vi "State_Machine.vi"(0 "Path In":path, 1 "Emergency":bool, 2 "Start Process":bool, 3 "Initialized":bool, 4 "Input Validated":bool, 5 "error in (no error)":errorcluster, 6 "Action":enum16{""}(ring), 7 "Running Done":bool, 9 "Process Complete":bool, 11 "Progressing":bool, 12 "Reset":bool, 13 "Powering Down":bool) -> (14 "Path Out":path, 15 "State":dbl, 16 "State String":string, 19 "error out":errorcluster)   [LabVIEW 2018]
panel:
  in  "Empty 2":bool
  in  "Empty1":bool
  out "_C_Powering_Down":bool
  out "_C_Empty_2":bool
  out "_C_Start_Process":bool
  out "_C_Empty_1":bool
  out "_C_Progressing":bool
  out "_C_Process Complete":bool
  out "_C_Running_Done":bool
  out "_C_Input_Validated":bool
  out "_C_Initialized":bool
  out "_C_emergency":bool
  out "_Powering Down":bool
  out "_Progressing Stage":bool
  out "_Completing Stage":bool
  out "_Running Stage":bool
  out "_Validating Input":bool
  out "_Initializing":bool
  out "_Idle":bool
  out "_Emergency":bool
  out "_Current_State":dbl
  # "~~~STATE MACHINE OUTPUT KEY~~~\n~~~ 1x Numeric & 1x Boolean ~~~\n(neg) - Emergency\n   All negative values\n(max) - Powering Down\n   All values above max\n0 -Idle\n1 - Initializing\n2 - Validating Input\n3 - Running Stage\n4 - Completing Stage\n5 - Progressing Stage\nBoolean - (T/F) Emergency Status"
  # "~~~INPUT CONDITIONS KEY~~~\n~~~ x10 Boolean Values~~~\n1 - Emergency\n2 - Start Process\n3 - Initialized\n4 - Input Validated\n5 - Running Done\n6 - Process Complete\n7 - Progressing (To next stage)\n8 - (Empty 1)\n9 - (Empty 2)\n10 - Powering Down"
  # "Local Variables (Used For Debugging)"
  # "State Lights"
  # "Condition Lights"
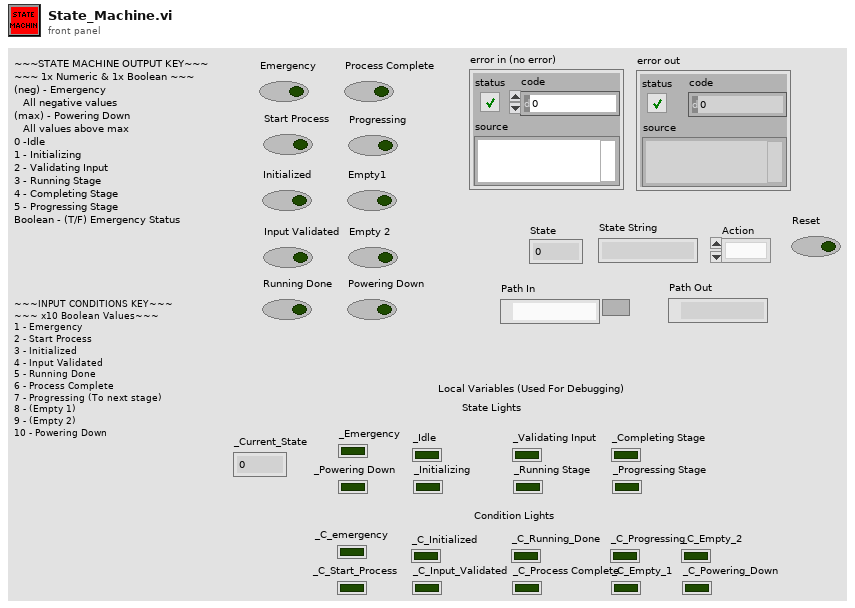
[diagram p1: front panel]
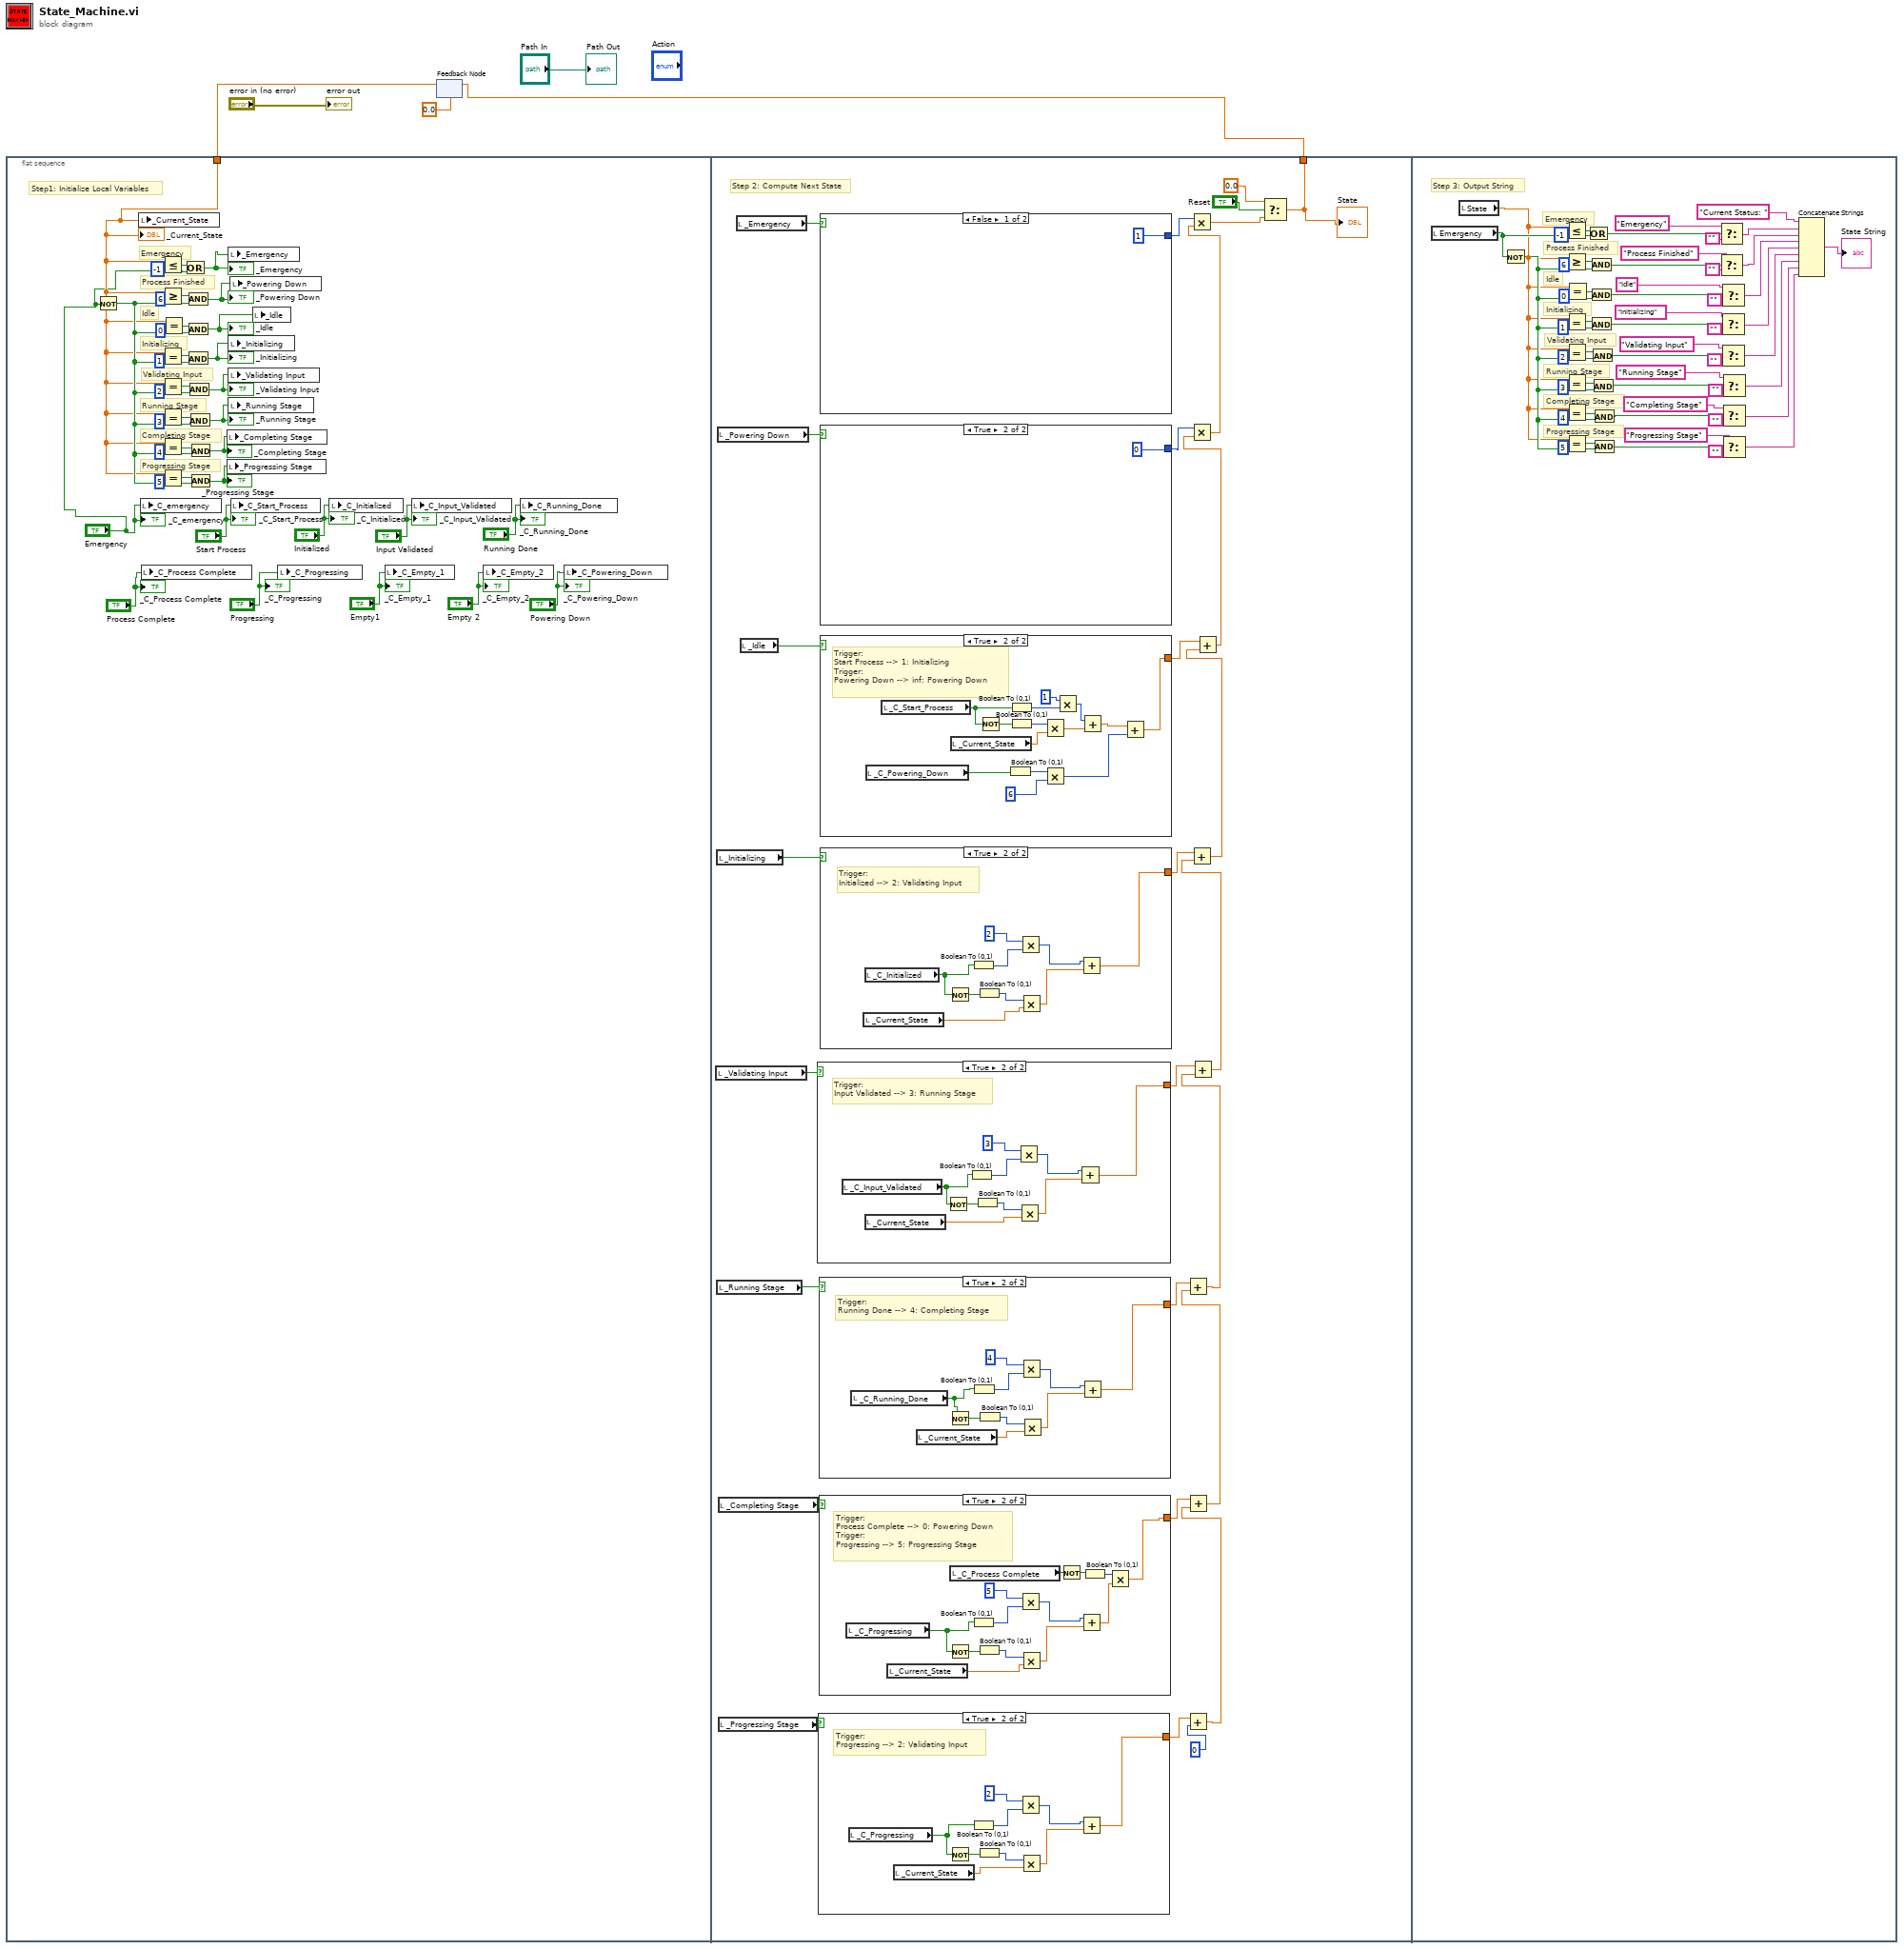
[diagram p0: block diagram]
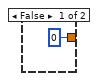
[diagram p2: hidden frame]
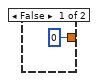
[diagram p3: hidden frame]
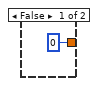
[diagram p4: hidden frame]
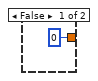
[diagram p5: hidden frame]
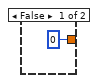
[diagram p6: hidden frame]
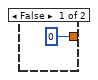
[diagram p7: hidden frame]
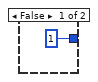
[diagram p8: hidden frame]
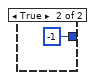
[diagram p9: hidden frame]
diagram:
  n1 = flat-sequence {
    tunnel: w4 -> [w16]
    tunnel: [w42] -> w1
    frame #0 {
      # "Step1: Initialize Local Variables"
      # "Emergency"
      # "Process Finished"
      # "Progressing Stage"
      # "Completing Stage"
      # "Running Stage"
      # "Validating Input"
      # "Initializing"
      # "Idle"
      n2 = Not(x="Emergency") -> (.not. x?=w30:bool)
      n3 = local write "_Current_State"(w16) -> ()
      n4 = local write "_C_emergency"("Emergency") -> ()
      n5 = local write "_C_Process Complete"("Process Complete") -> ()
      n6 = Less Or Equal?(x=w16, y=-1) -> (x <= y?=w19:bool)
      n7 = Greater Or Equal?(x=w16, y=6) -> (x >= y?=w17:bool)
      n8 = Equal?(x=w16, y=1) -> (x = y?=w32:bool)
      n9 = Equal?(x=w16, y=2) -> (x = y?=w33:bool)
      n10 = Equal?(x=w16, y=3) -> (x = y?=w34:bool)
      n11 = Equal?(x=w16, y=4) -> (x = y?=w35:bool)
      n12 = Equal?(x=w16, y=5) -> (x = y?=w21:bool)
      n13 = Equal?(x=w16, y=0) -> (x = y?=w31:bool)
      n14 = Or(x=w19, y="Emergency") -> (x .or. y?=w29:bool)
      "_Emergency" <- w29
      n15 = And(x=w17, y=w30) -> (x .and. y?=w28:bool)
      "_Powering Down" <- w28
      n16 = And(x=w31, y=w30) -> (x .and. y?=w27:bool)
      "_Idle" <- w27
      n17 = And(x=w32, y=w30) -> (x .and. y?=w26:bool)
      "_Initializing" <- w26
      n18 = And(x=w33, y=w30) -> (x .and. y?=w25:bool)
      "_Validating Input" <- w25
      n19 = And(x=w34, y=w30) -> (x .and. y?=w24:bool)
      "_Running Stage" <- w24
      n20 = And(x=w35, y=w30) -> (x .and. y?=w23:bool)
      "_Completing Stage" <- w23
      n21 = And(x=w21, y=w30) -> (x .and. y?=w22:bool)
      "_Progressing Stage" <- w22
      n22 = local write "_Completing Stage"(w23) -> ()
      n23 = local write "_Progressing Stage"(w22) -> ()
      n24 = local write "_Emergency"(w29) -> ()
      n25 = local write "_Initializing"(w26) -> ()
      n26 = local write "_Validating Input"(w25) -> ()
      n27 = local write "_Running Stage"(w24) -> ()
      n28 = local write "_Powering Down"(w28) -> ()
      n29 = local write "_C_Start_Process"("Start Process") -> ()
      n30 = local write "_Idle"(w27) -> ()
      n31 = local write "_C_Progressing"("Progressing") -> ()
      n32 = local write "_C_Initialized"("Initialized") -> ()
      n33 = local write "_C_Empty_1"("Empty1") -> ()
      n34 = local write "_C_Input_Validated"("Input Validated") -> ()
      n35 = local write "_C_Empty_2"("Empty 2") -> ()
      n36 = local write "_C_Running_Done"("Running Done") -> ()
      n37 = local write "_C_Powering_Down"("Powering Down") -> ()
      "_Current_State" <- w16
      "_C_emergency" <- "Emergency"
      "_C_Initialized" <- "Initialized"
      "_C_Input_Validated" <- "Input Validated"
      "_C_Running_Done" <- "Running Done"
      "_C_Process Complete" <- "Process Complete"
      "_C_Progressing" <- "Progressing"
      "_C_Empty_1" <- "Empty1"
      "_C_Start_Process" <- "Start Process"
      "_C_Empty_2" <- "Empty 2"
      "_C_Powering_Down" <- "Powering Down"
    }
    frame #1 {
      # "Step 2: Compute Next State"
      n38 = local read "_Validating Input"() -> (w65:bool)
      n39 = local read "_Initializing"() -> (w66:bool)
      n40 = local read "_Running Stage"() -> (w64:bool)
      n41 = local read "_Powering Down"() -> (w68:bool)
      n42 = local read "_Completing Stage"() -> (w63:bool)
      n43 = local read "_Progressing Stage"() -> (w62:bool)
      n44 = local read "_Emergency"() -> (w69:bool)
      n45 = local read "_Idle"() -> (w67:bool)
      n46 = case shown="True" w65 {
        tunnel: [0 w105] -> w52
        frame False {
        }
        frame True {
          # "Trigger:\nInput Validated --> 3: Running Stage"
          n47 = local read "_C_Input_Validated"() -> (w107:bool)
          n48 = local read "_Current_State"() -> (w106:dbl)
          n49 = Not(x=w107) -> (.not. x?=w113:bool)
          n50 = Boolean To (0,1)(Boolean=w107) -> (0, 1=w111:i16)
          n51 = Boolean To (0,1)(Boolean=w113) -> (0, 1=w110:i16)
          n52 = Multiply(x=3, y=w111) -> (x*y=w108:i32)
          n53 = Multiply(x=w110, y=w106) -> (x*y=w109:dbl)
          n54 = Add(x=w108, y=w109) -> (x+y=w105:dbl)
        }
      }
      n55 = case shown="True" w62 {
        tunnel: [0 w71] -> w49
        frame False {
        }
        frame True {
          # "Trigger:\nProgressing --> 2: Validating Input"
          n56 = local read "_C_Progressing"() -> (w73:bool)
          n57 = local read "_Current_State"() -> (w72:dbl)
          n58 = Not(x=w73) -> (.not. x?=w79:bool)
          n59 = Boolean To (0,1)(Boolean=w73) -> (0, 1=w77:i16)
          n60 = Boolean To (0,1)(Boolean=w79) -> (0, 1=w76:i16)
          n61 = Multiply(x=2, y=w77) -> (x*y=w74:i32)
          n62 = Multiply(x=w76, y=w72) -> (x*y=w75:dbl)
          n63 = Add(x=w74, y=w75) -> (x+y=w71:dbl)
        }
      }
      n64 = case shown="True" w64 {
        tunnel: [0 w95] -> w51
        frame False {
        }
        frame True {
          # "Trigger:\nRunning Done --> 4: Completing Stage"
          n65 = local read "_C_Running_Done"() -> (w97:bool)
          n66 = local read "_Current_State"() -> (w96:dbl)
          n67 = Not(x=w97) -> (.not. x?=w103:bool)
          n68 = Boolean To (0,1)(Boolean=w97) -> (0, 1=w101:i16)
          n69 = Boolean To (0,1)(Boolean=w103) -> (0, 1=w100:i16)
          n70 = Multiply(x=4, y=w101) -> (x*y=w98:i32)
          n71 = Multiply(x=w100, y=w96) -> (x*y=w99:dbl)
          n72 = Add(x=w98, y=w99) -> (x+y=w95:dbl)
        }
      }
      n73 = case shown="True" w63 {
        tunnel: [0 w86] -> w50
        frame False {
        }
        frame True {
          # "Trigger:\nProcess Complete --> 0: Powering Down\nTrigger:\nProgressing --> 5: Progressing Stage"
          n74 = local read "_C_Progressing"() -> (w85:bool)
          n75 = local read "_Current_State"() -> (w84:dbl)
          n76 = Not(x=w85) -> (.not. x?=w93:bool)
          n77 = local read "_C_Process Complete"() -> (w83:bool)
          n78 = Boolean To (0,1)(Boolean=w85) -> (0, 1=w91:i16)
          n79 = Boolean To (0,1)(Boolean=w93) -> (0, 1=w90:i16)
          n80 = Multiply(x=5, y=w91) -> (x*y=w88:i32)
          n81 = Multiply(x=w90, y=w84) -> (x*y=w89:dbl)
          n82 = Not(x=w83) -> (.not. x?=w82:bool)
          n83 = Add(x=w88, y=w89) -> (x+y=w87:dbl)
          n84 = Boolean To (0,1)(Boolean=w82) -> (0, 1=w81:i16)
          n85 = Multiply(x=w81, y=w87) -> (x*y=w86:dbl)
        }
      }
      n86 = case shown="False" w69 {
        tunnel: [1 -1] -> w61
        frame False {
        }
        frame True {
        }
      }
      n87 = case shown="True" w68 {
        tunnel: [1 0] -> w46
        frame False {
        }
        frame True {
        }
      }
      n88 = case shown="True" w67 {
        tunnel: [0 w130] -> w54
        frame False {
        }
        frame True {
          # "Trigger:\nStart Process --> 1: Initializing\nTrigger:\nPowering Down --> inf: Powering Down"
          n89 = local read "_C_Powering_Down"() -> (w128:bool)
          n90 = local read "_C_Start_Process"() -> (w137:bool)
          n91 = local read "_Current_State"() -> (w134:dbl)
          n92 = Not(x=w137) -> (.not. x?=w138:bool)
          n93 = Boolean To (0,1)(Boolean=w128) -> (0, 1=w127:i16)
          n94 = Boolean To (0,1)(Boolean=w137) -> (0, 1=w135:i16)
          n95 = Boolean To (0,1)(Boolean=w138) -> (0, 1=w133:i16)
          n96 = Multiply(x=w133, y=w134) -> (x*y=w132:dbl)
          n97 = Multiply(x=w127, y=6) -> (x*y=w125:i32)
          n98 = Multiply(x=1, y=w135) -> (x*y=w131:i32)
          n99 = Add(x=w131, y=w132) -> (x+y=w129:dbl)
          n100 = Add(x=w129, y=w125) -> (x+y=w130:dbl)
        }
      }
      n101 = case shown="True" w66 {
        tunnel: [0 w115] -> w53
        frame False {
        }
        frame True {
          # "Trigger:\nInitialized --> 2: Validating Input"
          n102 = local read "_Current_State"() -> (w117:dbl)
          n103 = local read "_C_Initialized"() -> (w116:bool)
          n104 = Not(x=w116) -> (.not. x?=w123:bool)
          n105 = Boolean To (0,1)(Boolean=w116) -> (0, 1=w121:i16)
          n106 = Boolean To (0,1)(Boolean=w123) -> (0, 1=w120:i16)
          n107 = Multiply(x=2, y=w121) -> (x*y=w118:i32)
          n108 = Multiply(x=w120, y=w117) -> (x*y=w119:dbl)
          n109 = Add(x=w118, y=w119) -> (x+y=w115:dbl)
        }
      }
      n110 = Add(x=w49, y=0) -> (x+y=w56:dbl)
      n111 = Add(x=w50, y=w56) -> (x+y=w57:dbl)
      n112 = Add(x=w51, y=w57) -> (x+y=w58:dbl)
      n113 = Add(x=w52, y=w58) -> (x+y=w59:dbl)
      n114 = Add(x=w53, y=w59) -> (x+y=w60:dbl)
      n115 = Add(x=w54, y=w60) -> (x+y=w47:dbl)
      n116 = Multiply(x=w46, y=w47) -> (x*y=w48:dbl)
      n117 = Multiply(x=w61, y=w48) -> (x*y=w45:dbl)
      n118 = Select(t=0.0, s="Reset", f=w45) -> (s? t:f=w42:dbl)
      "State" <- w42
    }
    frame #2 {
      # "Emergency"
      # "Process Finished"
      # "Progressing Stage"
      # "Completing Stage"
      # "Running Stage"
      # "Validating Input"
      # "Initializing"
      # "Idle"
      # "Step 3: Output String"
      n119 = local read "Emergency"() -> (w178:bool)
      n120 = local read "State"() -> (w148:dbl)
      n121 = Not(x=w178) -> (.not. x?=w179:bool)
      n122 = Less Or Equal?(x=w148, y=-1) -> (x <= y?=w182:bool)
      n123 = Greater Or Equal?(x=w148, y=6) -> (x >= y?=w180:bool)
      n124 = Equal?(x=w148, y=1) -> (x = y?=w186:bool)
      n125 = Equal?(x=w148, y=2) -> (x = y?=w187:bool)
      n126 = Equal?(x=w148, y=3) -> (x = y?=w188:bool)
      n127 = Equal?(x=w148, y=4) -> (x = y?=w189:bool)
      n128 = Equal?(x=w148, y=5) -> (x = y?=w184:bool)
      n129 = Equal?(x=w148, y=0) -> (x = y?=w185:bool)
      n130 = Or(x=w182, y=w178) -> (x .or. y?=w177:bool)
      n131 = And(x=w180, y=w179) -> (x .and. y?=w174:bool)
      n132 = And(x=w185, y=w179) -> (x .and. y?=w173:bool)
      n133 = And(x=w186, y=w179) -> (x .and. y?=w172:bool)
      n134 = And(x=w187, y=w179) -> (x .and. y?=w171:bool)
      n135 = And(x=w188, y=w179) -> (x .and. y?=w170:bool)
      n136 = And(x=w189, y=w179) -> (x .and. y?=w169:bool)
      n137 = And(x=w184, y=w179) -> (x .and. y?=w168:bool)
      n138 = Select(t="Emergency", s=w177, f="") -> (s? t:f=w144:string)
      n139 = Select(t="Process Finished", s=w174, f="") -> (s? t:f=w145:string)
      n140 = Select(t="Idle", s=w173, f="") -> (s? t:f=w146:string)
      n141 = Select(t="Initializing", s=w172, f="") -> (s? t:f=w149:string)
      n142 = Select(t="Validating Input", s=w171, f="") -> (s? t:f=w150:string)
      n143 = Select(t="Running Stage", s=w170, f="") -> (s? t:f=w151:string)
      n144 = Select(t="Completing Stage", s=w169, f="") -> (s? t:f=w152:string)
      n145 = Select(t="Progressing Stage", s=w168, f="") -> (s? t:f=w153:string)
      n146 = Concatenate Strings("Current Status: ", w144, w145, w146, w149, w150, w151, w152, w153) -> (→"State String":string)
    }
  }
  n147 = feedback #1(0.0) -> (w4:dbl)
  n148 = feedback-in #1(w1) -> ()
  "error out" <- "error in (no error)"
  "Path Out" <- "Path In"
